vi "Add CSM-VI.vi"(6 "Config Path":path, 8 "error in (no error)":errorcluster, 11 "CSM-VI":path) -> (0 "error out":errorcluster)   [LabVIEW 2017, in "CSM-Helper API with lvcsm Support.lvlib"]
uses:
  CSM-Helper API with lvcsm Support.lvlib
  4050c0ca-c03f-4557-9b57-a0dfa28f159e.vi
  210375e6-e1c9-4ab3-add6-b4e97a50608c.vi
  e1e95692-d4ce-4abb-8149-ad52922b776e.vi
  <vilib>/Utility/config.llb/Close Config Data.vi
  <vilib>/Utility/config.llb/Write Key.vi
  <vilib>/Utility/config.llb/Write Key (Double).vi
  <vilib>/Utility/config.llb/Write Key (I32).vi
  <vilib>/Utility/config.llb/Write Key (String).vi
  lvcsmFile/Path to lvcsm String.vi
  <vilib>/Utility/config.llb/Remove Key.vi
  <vilib>/Utility/config.llb/Get Key Names.vi
  <vilib>/Utility/Data Type/Get Type Information.vi
  <vilib>/Utility/Data Type/Get Array Information.vi
  <vilib>/Utility/config.llb/Write Key (Boolean).vi
  <vilib>/Utility/config.llb/Open Config Data.vi
  lvcsmFile/lvcsm File Path.vi
  API/Destroy.vi
  API/Update lvcsm Section in VI Description.vi
  Properties/Read Status.vi
  Properties/Read States.vi
  API/Create From Basic Refs.vi
  Utility/Is CSM Module - VIRef.vi
  Utility/CSM-Helper Utility.lvlib
  CSM-Helper.lvclass
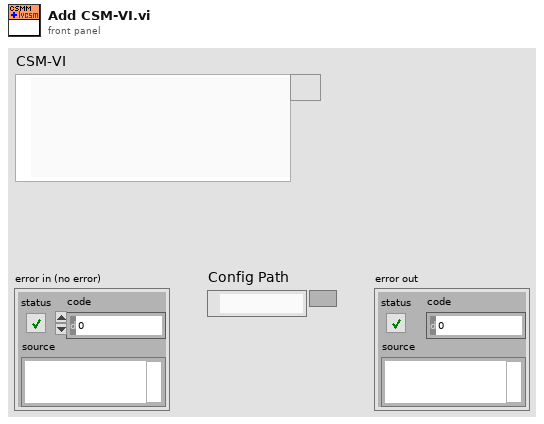
[diagram p1: front panel]
types:
  T1 = typedef "CSM-Helper Utility.lvlib/CSM Module Type.ctl" = enum16{"Not a CSM", "JKISM", "CSM"}
  T2 = typedef "CSM-Helper Utility.lvlib/CSM Basic Refs.ctl" = cluster{"VI":refnum<vi>, "While Loop":refnum<vi>, "Case Structure":refnum<vi>, "Parse State Queue":refnum<vi>, "Event Structure":refnum<vi>, "Type":T1, "InLvlibp":bool}
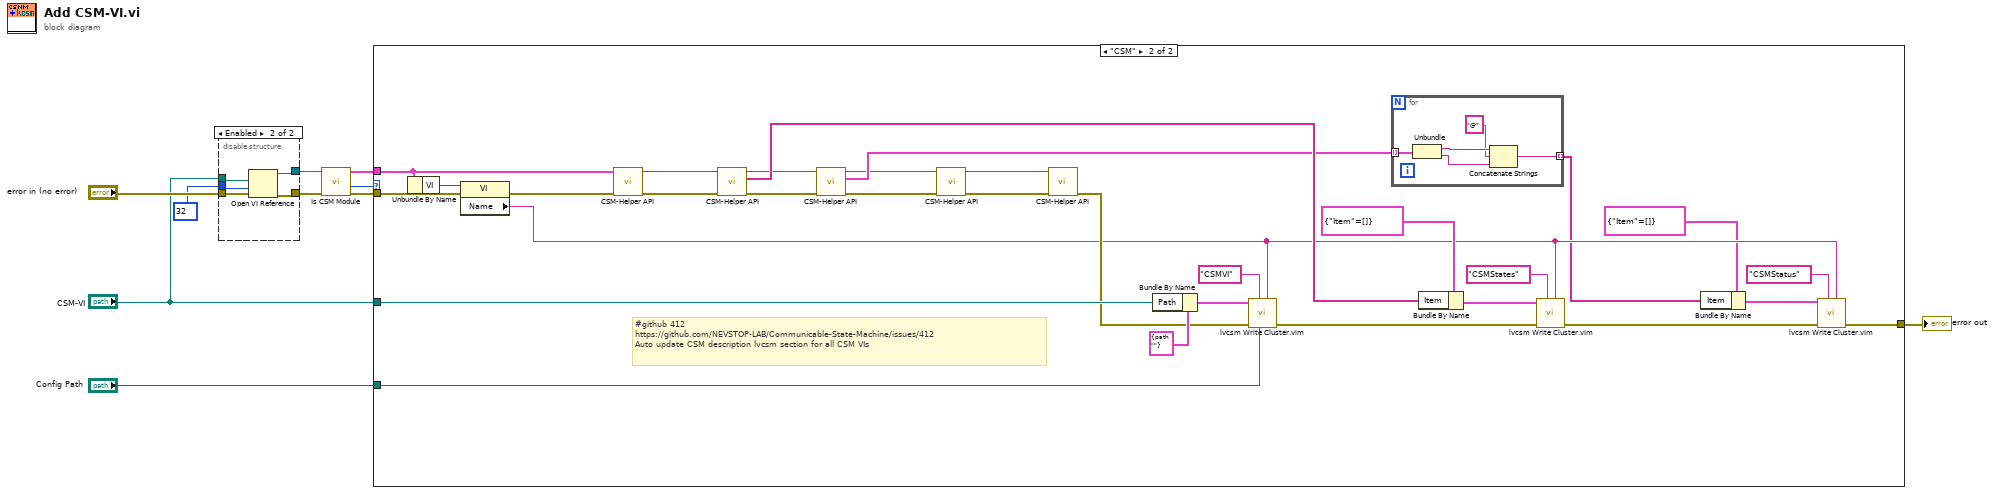
[diagram p0: block diagram]
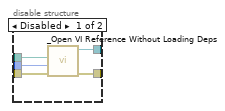
[diagram p2: hidden frame]
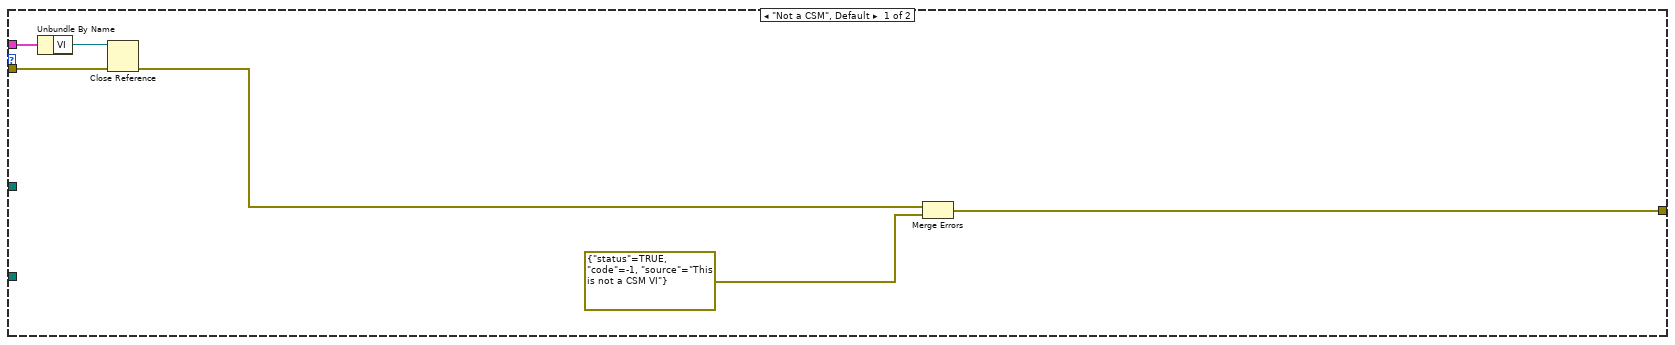
[diagram p3: hidden frame]
diagram:
  n1 = disable-structure shown="Enabled" {
    disable-tunnel: "error in (no error)" -> [w15 w19]
    disable-tunnel: [w14 w20] -> w7
    disable-tunnel: [w13 w16] -> w6
    disable-tunnel: "CSM-VI" -> [w12 w17]
    disable-tunnel: 32 ("options") -> [w11 w18]
    frame Disabled {
      n2 = call "_Open VI Reference Without Loading Deps.vi"("error in (no error)"=w15, "Options"=w11, "CSM-VI"=w12) -> ("error out"=w14:errorcluster, "VI Out"=w13:refnum<vi>)  [unwired: 7 in]
    }
    frame Enabled {
      n3 = Open VI Reference(vi path=w17, options=w18, error in (no error)=w19) -> (vi reference=w16:refnum<vi>, error out=w20:errorcluster)  [unwired: 3 in]
    }
  }
  n4 = call-poly "Is CSM Module.vi"("error in (no error)"=w7, "VIRef"=w6) -> ("error out"=w4:errorcluster, "CSMType"=w1:T1, "CSM Basic Refs"=w5:T2)  [unwired: 6 in, 1 out]
  n5 = case shown="\"CSM\"" w1 {
    tunnel: "Config Path" -> [_ w56]
    tunnel: [w22 w36] -> w8
    tunnel: "CSM-VI" -> [_ w53]
    tunnel: w4 -> [w26 w52]
    tunnel: w5 -> [w24 w50]
    frame "Not a CSM", Default {
      n6 = Unbundle By Name(w24) -> ("VI"=w23:refnum<vi>)
      n7 = Close Reference(reference=w23, error in (no error)=w26) -> (error out=w25:errorcluster)
      n8 = Merge Errors(w25, errorcluster {"status"=TRUE, "code"=-1, "source"="This is not a CSM VI"} ("error in")) -> (w22:errorcluster)
    }
    frame "CSM" {
      # "#github 412\nhttps://github.com/NEVSTOP-LAB/Communicable-State-Machine/issues/412 \nAuto update CSM description lvcsm section for all CSM VIs"
      n9 = Unbundle By Name(w50) -> ("VI"=w49:refnum<vi>)
      n10 = property class="VI"(reference=w49, error in=w52) -> (error out=w51:errorcluster, "Name"=w35:string)  [unwired: 1 out]
      n11 = call-poly "CSM-Helper API.vi"("error in (no error)"=w51, "CSM Basic Refs"=w50) -> ("error out"=w48:errorcluster, "CSM-Helper.lvclass"=w47:refnum<class "CSM-Helper.lvclass">)  [unwired: 8 in]
      n12 = call-poly "CSM-Helper API.vi"("error in (no error)"=w48, "CSM-Helper in"=w47) -> ("error out"=w40:errorcluster, "Value"=w43:string[], "CSM-Helper out"=w39:refnum<class "CSM-Helper.lvclass">)  [unwired: 7 in]
      n13 = call-poly "CSM-Helper API.vi"("error in (no error)"=w40, "CSM-Helper in"=w39) -> ("error out"=w30:errorcluster, "Array 3"=w32:cluster{"Status":string, "InState":string}[], "CSM-Helper out"=w29:refnum<class "CSM-Helper.lvclass">)  [unwired: 7 in]
      n14 = call-poly "CSM-Helper API.vi"("error in (no error)"=w30, "CSM-Helper in"=w29) -> ("error out"=w28:errorcluster, "CSM-Helper out"=w27:refnum<class "CSM-Helper.lvclass">)  [unwired: 8 in]
      n15 = call-poly "CSM-Helper API.vi"("error in (no error)"=w28, "CSM-Helper in"=w27) -> ("error out"=w41:errorcluster)  [unwired: 8 in, 1 out]
      n16 = Bundle By Name(cluster=cluster{"Path":path} {"Path"=path ""} ("Cluster 2"), "Path"=w53) -> (w57:cluster{"Path":path})
      n17 = call "lvcsm Write Cluster.vim"("Sub-section (\"\")"=w35, "Config Path"=w56, "Section"="CSMVI", "Error In"=w41, "Configuration"=w57) -> ("error out"=w44:errorcluster)  [unwired: 6 in]
      n18 = for {
        tunnel: w32 -> [w62] mode=indexing
        tunnel: [w58] -> w31 mode=indexing
        n19 = Unbundle(w62) -> ("Status"=w61:string, "InState"=w60:string)
        n20 = Concatenate Strings(w61, "@" ("string"), w60) -> (w58:string)
      }
      n21 = Bundle By Name(cluster=cluster{"Item":string[]} {"Item"=[]}, "Item"=w43) -> (w46:cluster{"Item":string[]})
      n22 = call "lvcsm Write Cluster.vim"("Sub-section (\"\")"=w35, "Section"="CSMStates", "Error In"=w44, "Configuration"=w46) -> ("error out"=w37:errorcluster)  [unwired: 7 in]
      n23 = Bundle By Name(cluster=cluster{"Item":string[]} {"Item"=[]}, "Item"=w31) -> (w33:cluster{"Item":string[]})
      n24 = call "lvcsm Write Cluster.vim"("Sub-section (\"\")"=w35, "Section"="CSMStatus", "Error In"=w37, "Configuration"=w33) -> ("error out"=w36:errorcluster)  [unwired: 7 in]
    }
  }
  "error out" <- w8
